vi "TV - Read actual velocity.vi"(2 "error in":errorcluster, 3 "Axis":i8=1 min=1 max=6 step=1, 4 "Address / Port":i16=1 min=1 max=31 step=1) -> (0 "error out":errorcluster, 1 "Read the controller status\nbyte in ASCII":string)   [LabVIEW 2014]
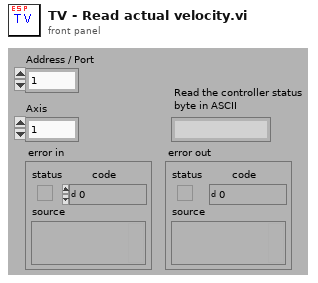
[diagram p1: front panel]
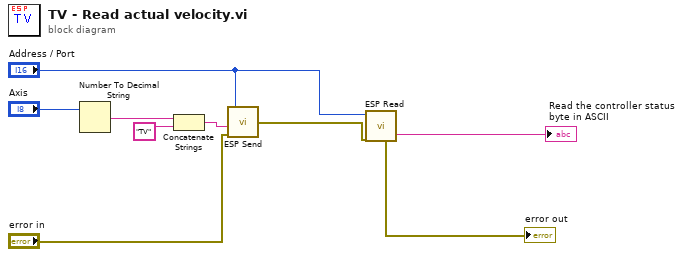
[diagram p0: block diagram]
diagram:
  n1 = Number To Decimal String(number="Axis") -> (decimal integer string=w8:string)  [unwired: 1 in]
  n2 = Concatenate Strings(w8, "TV" ("Substring")) -> (w6:string)
  n3 = call "ESP Send.vi"("Address / Port"="Address / Port", "Command String"=w6, "error in"="error in") -> ("error out"=w2:errorcluster)  [unwired: 5 in]
  n4 = call "ESP Read.vi"("Address / Port"="Address / Port", "error in"=w2) -> ("error out"=→"error out":errorcluster, "Response String"=→"Read the controller status\nbyte in ASCII":string)  [unwired: 5 in]
